vi "Calculate Contours.vi"(0 "mask image in":refnum<class "MSC Image.lvclass">, 5 "error in (no error)":errorcluster) -> (14 "mask image out":refnum<class "MSC Image.lvclass">, 15 "ROIs":T1[](array[typedef]) {"Type" items=["Point", "Line", "Rectangle", "Oval", "Freehand / Polygon"]}, 19 "error out":errorcluster)   [LabVIEW 2016, in "MSC Image.lvclass"]
doc: "Calculates contours of the input U8 image and returns them as ROIs with hierarchy information.\n\nThe hierarchy gives information which ROI contains other ROIs (children and parent system). Please dont delete or change the order of the ROIs if you want to use hierarchy."
uses:
  MSC Image.lvclass
  controls/ROI Type.ctl
  controls/Contour.ctl
  controls/Contour hierarchy.ctl
  controls/ROI.ctl
  Dependencies/x86/MSC I Process32.dll
  <userlib>/_OpenG.lib/array/array.llb/Search 1D Array (I32)__ogtk.vi
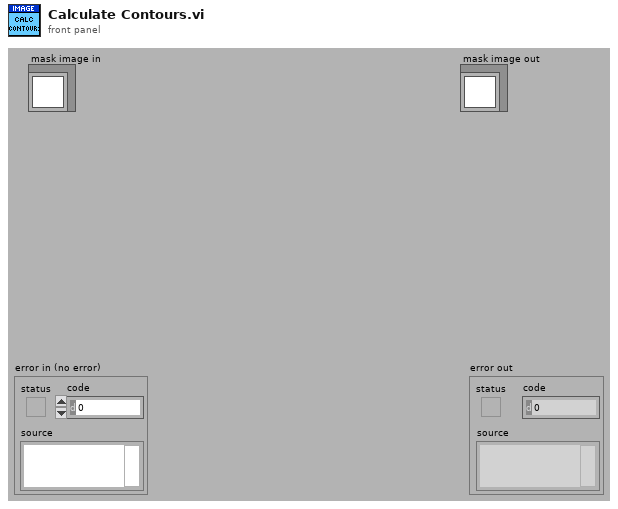
[diagram p1: front panel]
types:
  T1 = typedef "MSC Image.lvclass/ROI.ctl" = cluster{"Type":T2, "Parameters":dbl[], "Contour":T3, "Bounding Box":T3, "Contour Length":dbl, "ROI Area":dbl, "ROI Mean":dbl, "ROI Standard Deviation":dbl, "ROI Min":dbl, "ROI Max":dbl, "Hierarchy":T4, "Variant":variant, "Timestamp":timestamp}
  T2 = typedef "MSC Image.lvclass/ROI Type.ctl" = u16
  T3 = typedef "MSC Image.lvclass/Contour.ctl" = cluster{"x":i16, "y":i16}[]
  T4 = typedef "MSC Image.lvclass/Contour hierarchy.ctl" = cluster{"parent ID":i32, "children IDs":dbl[], "level":i32}
  T5 = typedef "Image.ctl" = cluster{"Pointer":u64, "Size":T6, "Image Type":T7, "Time Stamp":timestamp, "Variant":variant}
  T6 = typedef "Size.ctl" = cluster{"Cols":i32, "Rows":i32}
  T7 = typedef "Image Type.ctl" = i32
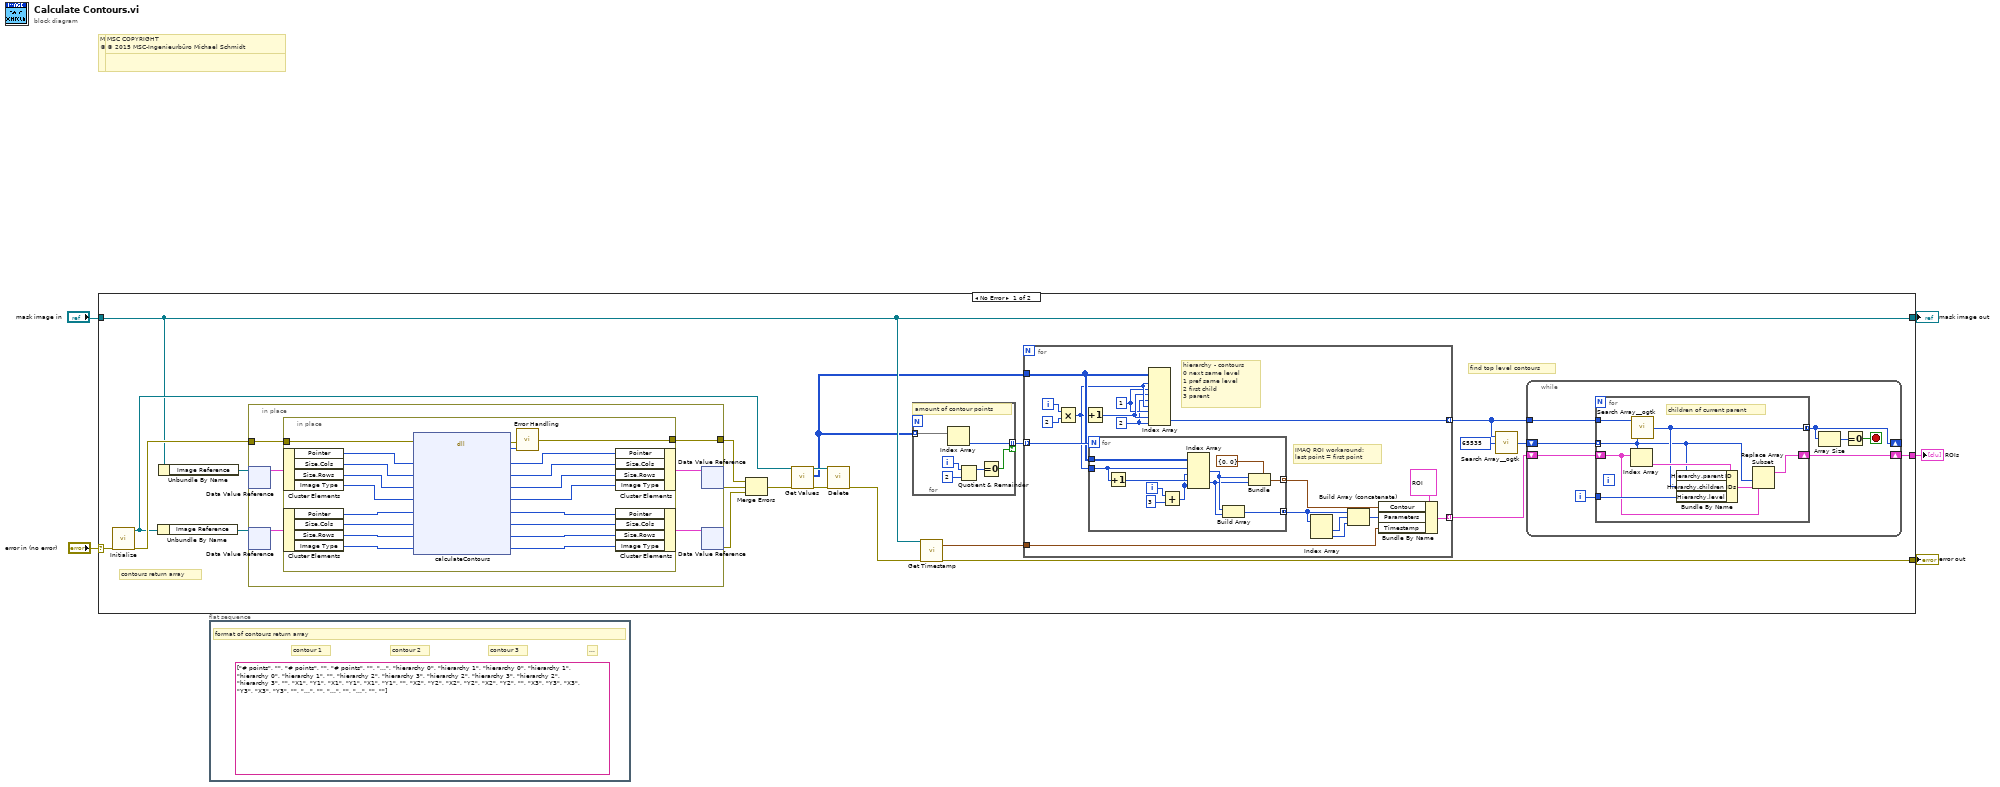
[diagram p0: block diagram]
diagram:
  # "MSC COPYRIGHT\n© 2016 MSC-Ingenieurbüro Michael Schmidt"
  # "MSC COPYRIGHT\n© 2016 MSC-Ingenieurbüro Michael Schmidt"
  # "MSC COPYRIGHT\n© 2015 MSC-Ingenieurbüro Michael Schmidt"
  # "MSC COPYRIGHT\n© 2015 MSC-Ingenieurbüro Michael Schmidt"
  n1 = case shown="No Error" "error in (no error)" {
    selector: "error in (no error)" -> [w24 w105]
    tunnel: [w8 w105] -> w4
    tunnel: [w13 w104] -> w2
    tunnel: "mask image in" -> [w13 w104]
    tunnel: [w6 _] -> w1
    frame No Error {
      # "contours return array"
      # "find top level contours"
      n2 = call "Initialize.vi"("error in (no error)"=w24) -> ("image out"=w19:refnum<class "MSC Image.lvclass">, "error out"=w25:errorcluster)  [unwired: 17 in]
      n3 = Unbundle By Name(w19) -> ("Image Reference"=w26:refnum<data-value>)
      n4 = Unbundle By Name(w13) -> ("Image Reference"=w27:refnum<data-value>)
      n5 = in-place {
        in-place-border: w25 -> [w81]
        in-place-border: [w80] -> w21
        n6 = in-place-dvr #1(w27) -> (w82:T5)  [unwired: 1 out]
        n7 = in-place-dvr #2(w26) -> (w79:T5)  [unwired: 1 out]
        n8 = in-place {
          in-place-border: w81 -> [w93]
          in-place-border: [w88] -> w80
          n9 = in-place-cluster #3(w82) -> ("Pointer"=w103:u64, "Size.Cols"=w102:i32, "Size.Rows"=w101:i32, "Image Type"=w100:T7)
          n10 = in-place-cluster #4(w79) -> ("Pointer"=w99:u64, "Size.Cols"=w98:i32, "Size.Rows"=w97:i32, "Image Type"=w96:T7)
          n11 = dll-call lib="C:/Users/MSC/LabVIEW Projekte/LV 2014/MSC I-Process/user.lib/MSC-I Process/Dependencies/x86/MSC I Process*.dll" fn="calculateContours"(error in=w93, "pointer"=w103, "cols"=w102, "rows"=w101, "type"=w100, "pointerCont"=w99, "colsCont"=w98, "rowsCont"=w97, "typeCont"=w96) -> (error out=w94:errorcluster, "error"=w95:i32, "pointer"=w92:u64, "cols"=w91:i32, "rows"=w90:i32, "type"=w89:i32, "pointerCont"=w87:u64, "colsCont"=w86:i32, "rowsCont"=w85:i32, "typeCont"=w84:i32)  [unwired: 2 in, 1 out]
          n12 = call "Error Handling.vi"("error in (no error)"=w94, "return type"=w95) -> ("error out"=w88:errorcluster)  [unwired: 12 in, 1 out]
          n13 = in-place-cluster #3("Pointer"=w92, "Size.Cols"=w91, "Size.Rows"=w90, "Image Type"=w89) -> (w83:T5)
          n14 = in-place-cluster #4("Pointer"=w87, "Size.Cols"=w86, "Size.Rows"=w85, "Image Type"=w84) -> (w78:T5)
        }
        n15 = in-place-dvr #1(w83) -> (w23:errorcluster)  [unwired: 1 out]
        n16 = in-place-dvr #2(w78) -> (w22:errorcluster)  [unwired: 1 out]
      }
      n17 = Merge Errors(w21, w23, w22) -> (w20:errorcluster)
      n18 = call-dynamic "Get Values.vi"("image in"=w19, "error in (no error)"=w20) -> ("image out"=w18:refnum<class "MSC Image.lvclass">, "imageData U16"=w12:u16[][], "error out"=w17:errorcluster)  [unwired: 10 in, 5 out]
      n19 = call-dynamic "Delete.vi"("image in"=w18, "error in (no error)"=w17) -> ("error out"=w14:errorcluster)  [unwired: 17 in]
      n20 = for {
        tunnel: w12 -> [w77] mode=indexing
        tunnel: [w73] -> w16 mode=indexing if=w72
        i -> [w76]
        # "amount of contour points"
        n21 = Index Array(array=w77) -> (element=w73:u16)  [unwired: 1 in]
        n22 = Quotient & Remainder(x=w76, y=2) -> (x-y*floor(x/y)=w74:i32)  [unwired: 1 out]
        n23 = Equal To 0?(x=w74) -> (x = 0?=w72:bool)
      }
      n24 = call-dynamic "Get Timestamp.vi"("image in"=w13, "error in (no error)"=w14) -> ("Time Stamp"=w15:timestamp, "error out"=w8:errorcluster)  [unwired: 15 in, 1 out]
      n25 = for {
        tunnel: w16 -> [w60] mode=indexing
        tunnel: w12 -> [w49]
        tunnel: [w55] -> w9 mode=indexing
        tunnel: w15 -> [w50]
        tunnel: [w44] -> w7 mode=indexing
        i -> [w59]
        w45 = 2 ("disabled index (col)")
        w46 = 1 ("disabled index (col)")
        # "hierarchy - contours\n0 next same level\n1 pref same level\n2 first child\n3 parent"
        # "IMAQ ROI workaround:\nlast point = first point"
        n26 = Multiply(x=w59, y=2) -> (x*y=w48:i32)
        n27 = Increment(x=w48) -> (x+1=w47:i32)
        n28 = for {
          N: w60 -> [_]
          tunnel: w48 -> [w70]
          tunnel: w49 -> [w71]
          tunnel: [w67] -> w56 mode=indexing
          tunnel: [w64] -> w52 mode=concatenating
          i -> [w63]
          n29 = Increment(x=w70) -> (x+1=w69:i32)
          n30 = Add(x=w63, y=3) -> (x+y=w62:i32)
          n31 = Index Array(array=w71, index (row) #1=w70, index (col) #1=w62, index (row) #2=w69, index (col) #2=w62) -> (element #1=w66:u16, element #2=w65:u16)
          n32 = Build Array(w66, w65) -> (w64:u16[])
          n33 = Bundle(cluster=cluster{"x":i16, "y":i16} {"x"=0, "y"=0} ("point"), "x"=w66, "y"=w65) -> (w67:cluster{"x":i16, "y":i16})
        }
        n34 = Index Array(array=w49, index (row) #1=w48, index (col) #1=w46, index (row) #2=w47, index (col) #2=w45, index (row) #3=w48, index (col) #3=w46, index (row) #4=w47, index (col) #4=w45) -> (element #4=w44:u16)  [unwired: 3 out]
        n35 = Index Array(array=w52) -> (element #1=w53:u16, element #2=w54:u16)  [unwired: 2 in]
        n36 = Build Array (concatenate)(w52, w53, w54) -> (w51:u16[])
        n37 = Bundle By Name(cluster=T1 {"Type"=4, "Parameters"=[], "Contour"=[], "Bounding Box"=[], "Contour Length"=0.0, "ROI Area"=0.0, "ROI Mean"=0.0, "ROI Standard Deviation"=0.0, "ROI Min"=0.0, "ROI Max"=0.0, "Hierarchy"={"parent ID"=0, "children IDs"=[], "level"=0}, "Variant"=variant, "Timestamp"=timestamp(0 s since 1904-01-01)} ("ROI"), "Contour"=w56, "Parameters"=w51, "Timestamp"=w50) -> (w55:T1)
      }
      n38 = call-poly <userlib>:"Search Array__ogtk.vi"("Array"=w7, "Element Data"=65535) -> ("Indices of Elements"=w10:i32[])  [unwired: 7 in]
      n39 = while {
        tunnel: w7 -> [w34]
        shift-right: [w30] -> _
        shift-left: w10 -> [w35]
        shift-right: [w29] -> w6
        shift-left: w9 -> [w28]
        i -> [w31]
        stop <- w32 stop-if-true
        n40 = for {
          tunnel: w35 -> [w38] mode=indexing
          tunnel: w34 -> [w43]
          tunnel: w31 -> [w40]
          tunnel: [w41] -> w30 mode=concatenating
          shift-right: [w39] -> w29
          shift-left: w28 -> [w36]
          # "children of current parent"
          n41 = Index Array(array=w36, index=w38) -> (element=w42:T1)
          n42 = call-poly <userlib>:"Search Array__ogtk.vi"("Array"=w43, "Element Data"=w38) -> ("Indices of Elements"=w41:i32[])  [unwired: 7 in]
          n43 = Bundle By Name(cluster=w42, "Hierarchy.parent ID"=w38, "Hierarchy.children IDs"=w41, "Hierarchy.level"=w40) -> (w37:T1)
          n44 = Replace Array Subset(array=w36, new element=w37, index=w38) -> (w39:T1[])
        }
        n45 = Array Size(array=w30) -> (size(s)=w33:i32)
        n46 = Equal To 0?(x=w33) -> (x = 0?=w32:bool)
      }
    }
    frame Error {
    }
  }
  "error out" <- w4
  "mask image out" <- w2
  "ROIs" <- w1
  n47 = flat-sequence {
    frame #0 {
      (unwired) string[][] [["# points", "", "# points", "", "# points", "", "..."], ["hierarchy 0", "hierarchy 1", "hierarchy 0", "hierarchy 1", "hierarchy 0", "hierarchy 1", ""], ["hierarchy 2", "hierarchy 3", "hierarchy 2", "hierarchy 3", "hierarchy 2", "hierarchy 3", ""], ["X1", "Y1", "X1", "Y1", "X1", "Y1", ""], ["X2", "Y2", "X2", "Y2", "X2", "Y2", ""], ["X3", "Y3", "X3", "Y3", "X3", "Y3", ""], ["...", "", "...", "", "...", "", ""]]
      # "..."
      # "contour 3"
      # "contour 2"
      # "contour 1"
      # "format of contours return array"
    }
  }
